vi "Send.vi"(6 "Timeout ms (1000)":i32=1000, 8 "Error In":errorcluster, 10 "Value":variant, 11 "Sender Ref.":refnum<class "Sender.lvclass">) -> (0 "Error Out":errorcluster, 3 "Sender Ref.":refnum<class "Sender.lvclass">)   [LabVIEW 2020, in "RemoteVariables.lvlib" / "Sender.lvclass"]
uses:
  Sender.lvclass
  Sender.lvclass/Sender.ctl
  RawData.ctl
  RemoteVariables.lvlib
  UDP/UDP.lvclass
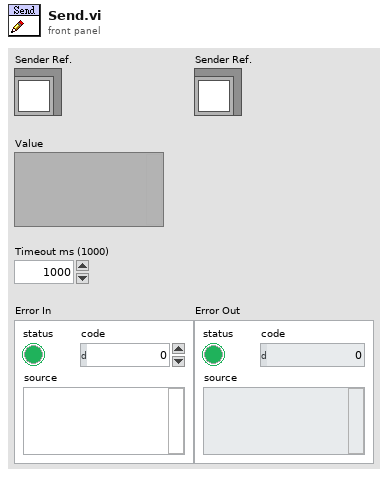
[diagram p1: front panel]
types:
  T1 = typedef "RemoteVariables.lvlib/RawData.ctl" = cluster{"Type string":i16[], "Data string":string}
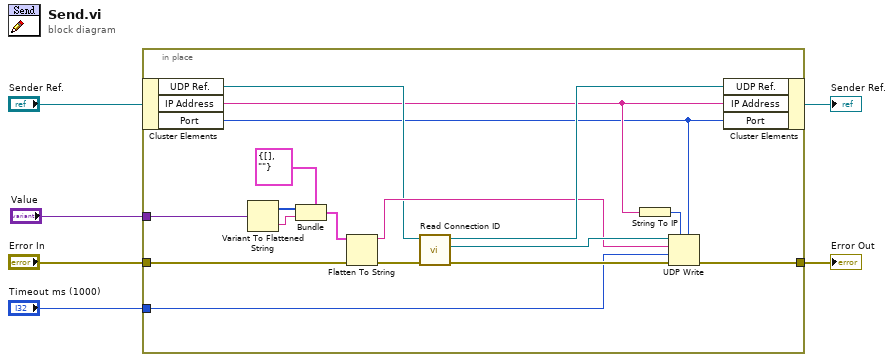
[diagram p0: block diagram]
diagram:
  n1 = in-place {
    in-place-border: "Value" -> [w20]
    in-place-border: "Error In" -> [w16]
    in-place-border: "Timeout ms (1000)" -> [w11]
    in-place-border: [w10] -> w2
    n2 = in-place-cluster #1("Sender Ref.") -> ("UDP Ref."=w12:refnum<class "UDP.lvclass">, "IP Address"=w9:string, "Port"=w7:u16)
    n3 = Variant To Flattened String(Variant=w20) -> (data string=w17:string, 1:w18:i16[])
    n4 = Bundle(cluster=T1 {"Type string"=[], "Data string"=""} ("RawData"), "Type string"=w18, "Data string"=w17) -> (w15:T1)
    n5 = Flatten To String(anything=w15, error in (no error)=w16) -> (data string=w13:string, error out=w14:errorcluster)  [unwired: 2 in, 1 out]
    n6 = call "Read Connection ID.vi"("error in (no error)"=w14, "UDP in"=w12) -> ("error out"=w21:errorcluster, "UDP Connection ID"=w22:refnum<k16>, "UDP out"=w23:refnum<class "UDP.lvclass">)  [unwired: 7 in]
    n7 = String To IP(1:w9) -> (0:w8:u32)
    n8 = UDP Write(address=w8, port or service name=w7, connection ID=w22, data in=w13, 8:w21, 9:w11) -> (error out=w10:errorcluster)  [unwired: 1 out]
    n9 = in-place-cluster #1("UDP Ref."=w23, "IP Address"=w9, "Port"=w7) -> (→"Sender Ref.":refnum<class "Sender.lvclass">)
  }
  "Error Out" <- w2
